vi "DSF.Shared.Configuration.Transfer.Set Direction.vi"(8 "error in (no error)":errorcluster, 10 "Direction":T1, 11 "Transfer Configuration in":refnum<class "DSF.Shared.Configuration.Transfer.lvclass">) -> (0 "error out":errorcluster, 3 "Transfer Configuration out":refnum<class "DSF.Shared.Configuration.Transfer.lvclass">)   [LabVIEW 2016, in "DSF.Shared.lvlib" / "DSF.Shared.Configuration.Transfer.lvclass"]
uses:
  DSF.Shared.Configuration.Transfer.lvclass
  Typedefs/DSF.Shared.Typedefs.Direction.ctl
  DSF.Shared.Configuration.Transfer.lvclass/DSF.Shared.Configuration.Transfer.ctl
  DSF.Shared.lvlib
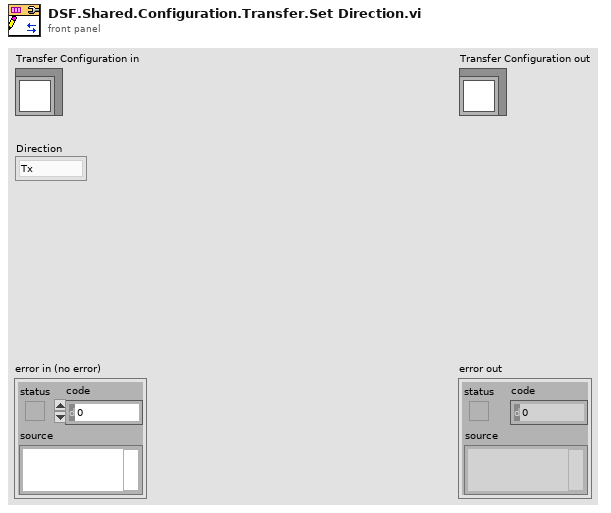
[diagram p1: front panel]
types:
  T1 = typedef "DSF.Shared.lvlib/DSF.Shared.Typedefs.Direction.ctl" = enum16{"Tx", "Rx"}
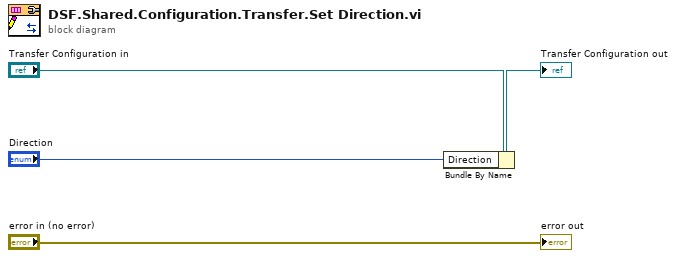
[diagram p0: block diagram]
diagram:
  n1 = Bundle By Name(cluster="Transfer Configuration in", "Direction"="Direction") -> (→"Transfer Configuration out":refnum<class "DSF.Shared.Configuration.Transfer.lvclass">)
  "error out" <- "error in (no error)"
